vi "ds set monitor baud rate.vi"(10 "baud_mode":u32, 11 "ds_handle":u32) -> (2 "function return":i32, 3 "ds_handle out":u32)   [LabVIEW 2019, in "apdm.lvlib"]
doc: "APDM_EXPORT int apdm_ds_set_monitor_baud_rate(apdm_device_handle_t ds_handle, const uint32_t baud_mode);"
uses:
  apdm.lvlib
  Lee Lab/CP FES Walking 2018/Code/Working/LabVIEW/apdm.dll
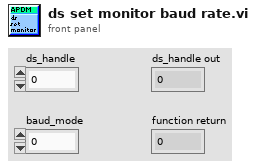
[diagram p1: front panel]
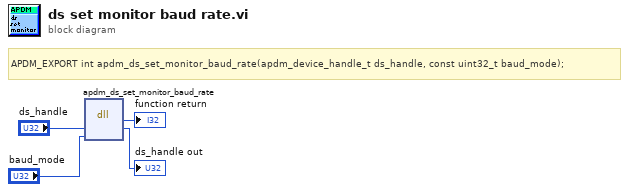
[diagram p0: block diagram]
diagram:
  # "APDM_EXPORT int apdm_ds_set_monitor_baud_rate(apdm_device_handle_t ds_handle, const uint32_t baud_mode);"
  n1 = dll-call lib="C:/Users/jfalesi/Dropbox/Lee Lab/CP FES Walking 2018/Code/Working/LabVIEW/apdm.*" fn="apdm_ds_set_monitor_baud_rate"("ds_handle"="ds_handle", "baud_mode"="baud_mode") -> (→"function return":i32, "ds_handle"=→"ds_handle out":u32)  [unwired: 4 in, 2 out]
